vi "Close AI.vi"(8 "error in (no error)":errorcluster, 11 "PXIe 6363 in":refnum<class "PXIe 6363.lvclass">) -> (0 "error out":errorcluster, 3 "PXIe 6363 out":refnum<class "PXIe 6363.lvclass">)   [LabVIEW 2021, in "DAQ Hardware.lvlib" / "PXIe 6363.lvclass"]
uses:
  PXIe 6363.lvclass
  PXIe 6363.lvclass/PXIe 6363.ctl
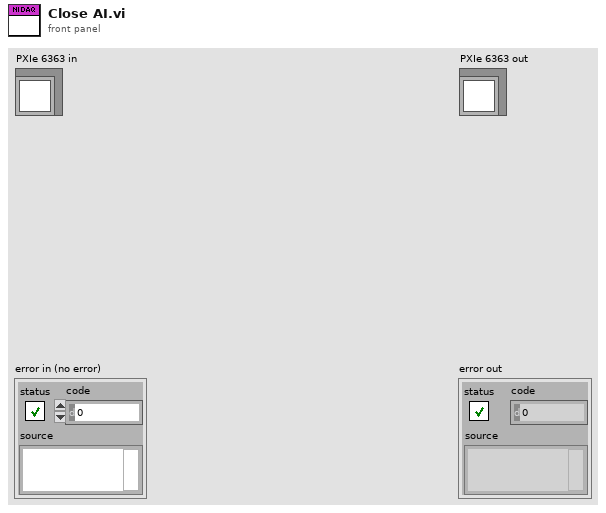
[diagram p1: front panel]
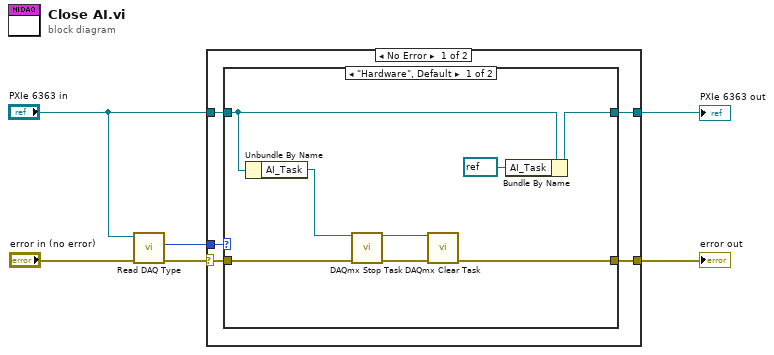
[diagram p0: block diagram]
diagram:
  n1 = call-dynamic "Read DAQ Type.vi"("error in (no error)"="error in (no error)", "PXIe 6363 in"="PXIe 6363 in") -> ("error out"=w5:errorcluster, "DAQ Type"=w4:enum16{"Hardware", "Simulation"})  [unwired: 7 in, 1 out]
  n2 = case shown="No Error" w5 {
    selector: w5 -> [w9 w22]
    tunnel: w4 -> [w11 _]
    tunnel: "PXIe 6363 in" -> [w10 w23]
    tunnel: [w8 w23] -> w2
    tunnel: [w7 w22] -> w1
    frame No Error {
      n3 = case shown="\"Hardware\", Default" w11 {
        tunnel: w10 -> [w15 w21]
        tunnel: w9 -> [w17 w20]
        tunnel: [w13 w21] -> w8
        tunnel: [w14 w20] -> w7
        frame "Hardware", Default {
          n4 = Unbundle By Name(w15) -> ("AI_Task"=w19:refnum<k21>)
          n5 = call <vilib>:"DAQmx Stop Task.vi"("task/channels in"=w19, "error in"=w17) -> ("task out"=w18:refnum<k21>, "error out"=w16:errorcluster)  [unwired: 12 in]
          n6 = call <vilib>:"DAQmx Clear Task.vi"("task in"=w18, "error in"=w16) -> ("error out"=w14:errorcluster)  [unwired: 13 in]
          n7 = Bundle By Name(cluster=w15, "AI_Task"=refnum<k21> refnum ("AI Task")) -> (w13:refnum<class "PXIe 6363.lvclass">)
        }
        frame "Simulation" {
        }
      }
    }
    frame Error {
    }
  }
  "error out" <- w1
  "PXIe 6363 out" <- w2
